vi "SharedTimer.vi"(1 "Write?":bool, 2 "TimerInput":T1) -> (0 "Timer":T1)   [LabVIEW 2010, in "Player.lvlib"]
uses:
  Player.lvlib
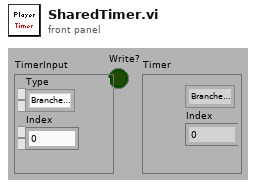
[diagram p1: front panel]
types:
  T1 = cluster{"Index":u16, "Type":enum8{"Branched Timer", "NXT Timer"}}
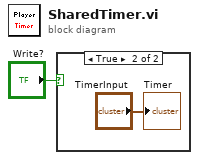
[diagram p0: block diagram]
diagram:
  n1 = case shown="True" "Write?" {
    frame False {
    }
    frame True {
      "Timer" <- "TimerInput"
    }
  }
